vi "Signal_generator.vi"() -> ()   [LabVIEW 2023]
uses:
  <vilib>/measure/NI_MABase.lvlib
panel:
  out "Waveform Chart":waveform(dbl)(graph)
  out "Waveform Graph":waveform(dbl)(graph)
  out "signal out":waveform(dbl)
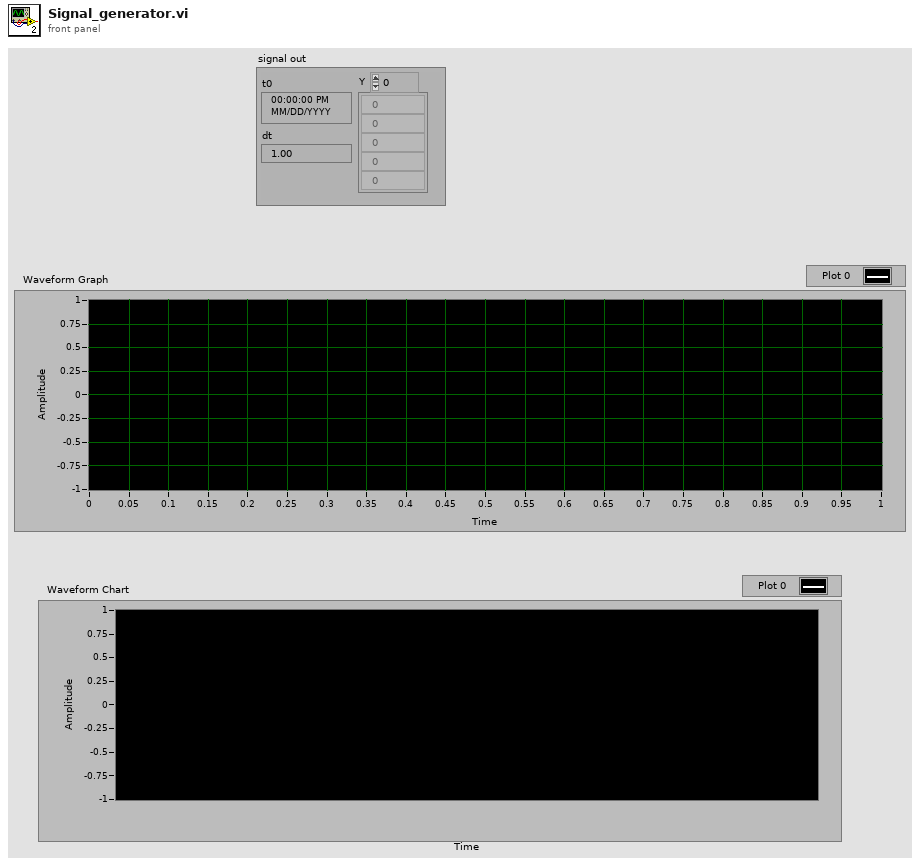
[diagram p1: front panel]
types:
  T1 = enum16{"Sine Wave", "Triangle Wave", "Square Wave", "Sawtooth Wave"}
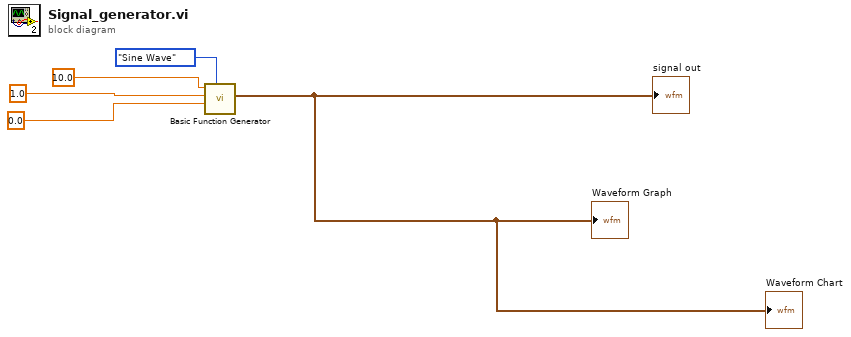
[diagram p0: block diagram]
diagram:
  n1 = call <vilib>:"Basic Function Generator.vi"("signal type"=T1."Sine Wave", "phase"=0.0, "amplitude"=1.0, "frequency"=10.0) -> ("signal out"=→"signal out" →"Waveform Graph" →"Waveform Chart":waveform(dbl))  [unwired: 5 in, 2 out]
